vi "CoriEngine.vi"(0 "object in":refnum<class "CoriFlowBFS1Plus.lvclass">, 2 "Sample Rate (Hz)":dbl=10.0 format="%#_13g", 5 "error in (no error)":errorcluster) -> (14 "object out":refnum<class "CoriFlowBFS1Plus.lvclass">, 19 "error out":errorcluster)   [LabVIEW 2021, in "CoriFlowBFS1Plus.lvclass"]
uses:
  CoriFlowBFS1Plus.lvclass
  CoriFlowBFS1Plus.lvclass/CoriFlowBFS1Plus.ctl
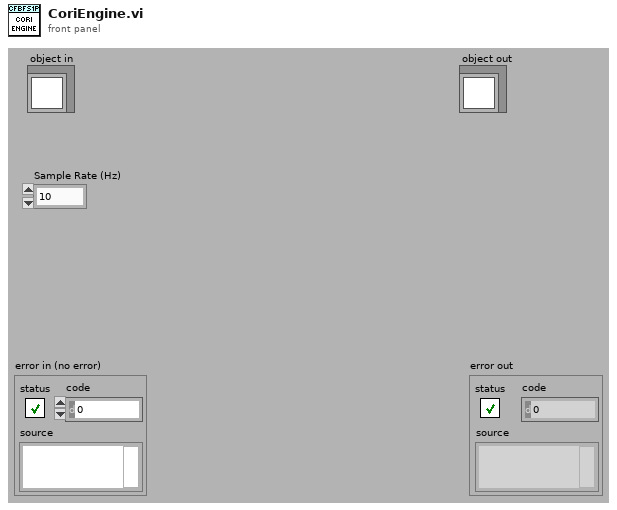
[diagram p1: front panel]
types:
  T1 = cluster{"Message":string, "Message Data":variant}
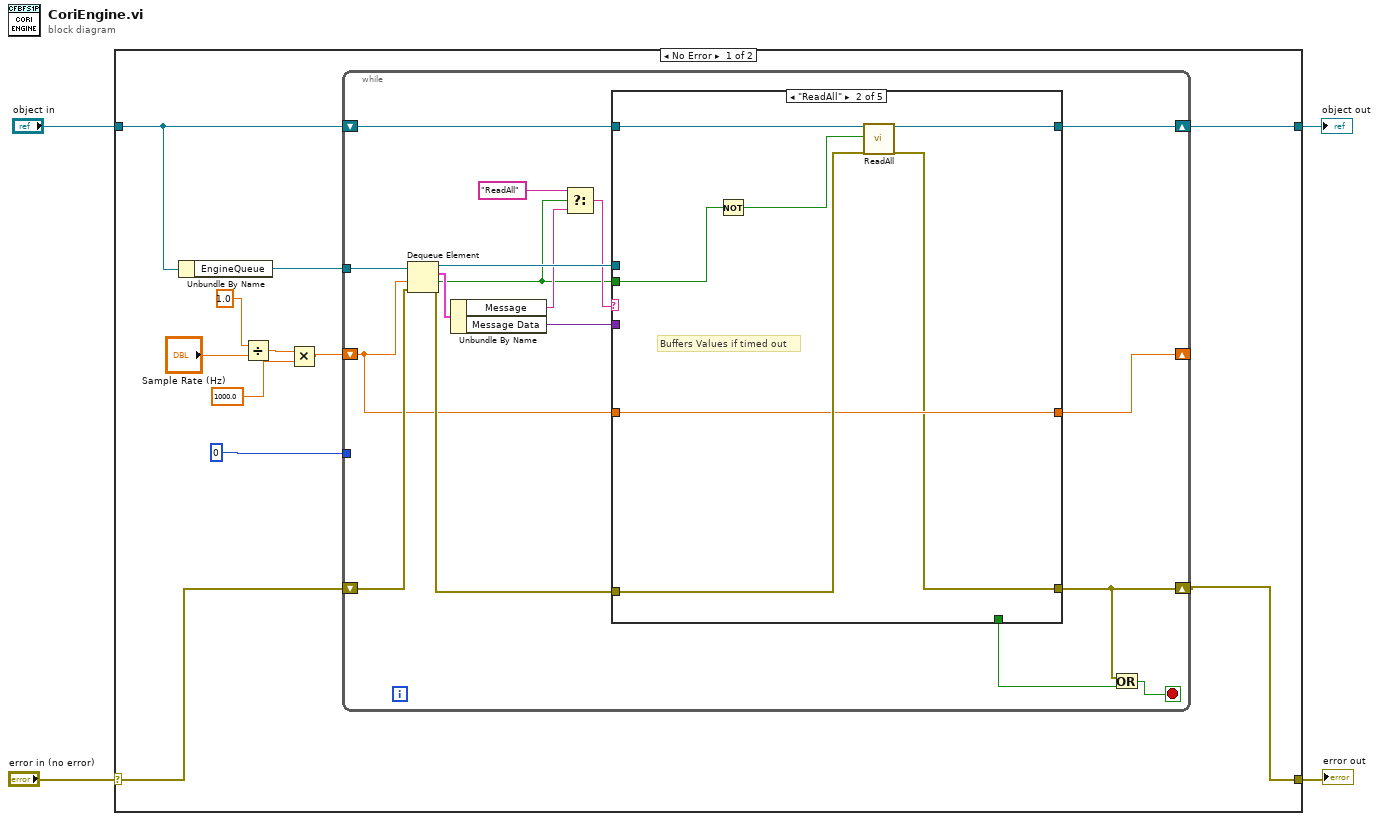
[diagram p0: block diagram]
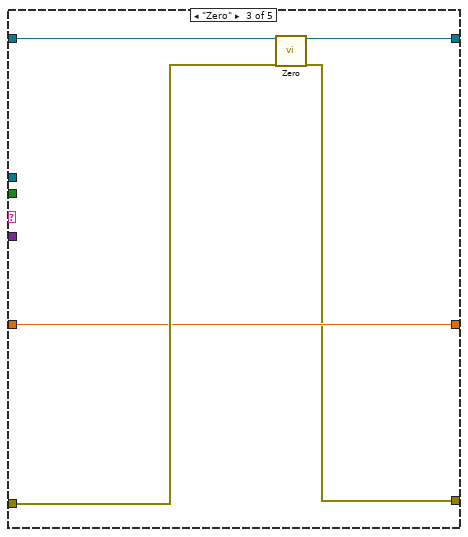
[diagram p3: hidden frame]
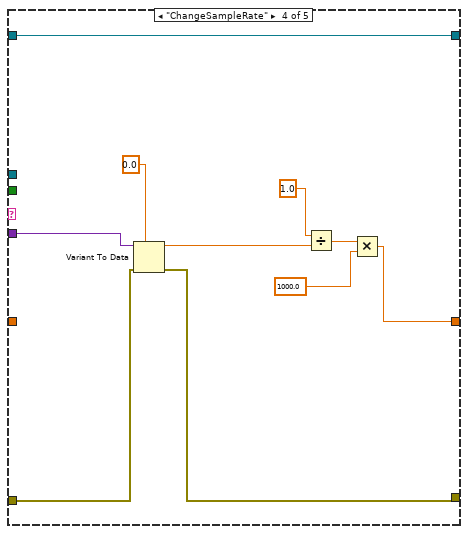
[diagram p4: hidden frame]
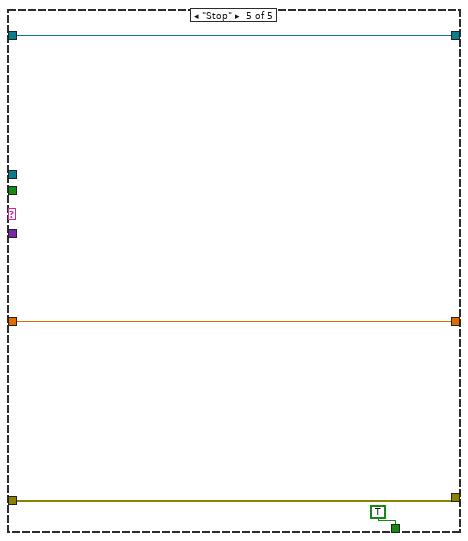
[diagram p5: hidden frame]
diagram:
  n1 = case shown="No Error" "error in (no error)" {
    selector: "error in (no error)" -> [w7 w63]
    tunnel: [w6 w63] -> w3
    tunnel: [w14 w62] -> w1
    tunnel: "object in" -> [w15 w62]
    frame No Error {
      n2 = Unbundle By Name(w15) -> ("EngineQueue"=w5:refnum<queue>)
      n3 = Divide(x=1.0, y="Sample Rate (Hz)") -> (x/y=w10:dbl)
      n4 = Multiply(x=w10, y=1000.0) -> (x*y=w8:dbl)
      n5 = while {
        shift-right: [w24] -> w14
        shift-left: w15 -> [w25]
        tunnel: w5 -> [w32]
        shift-right: [w27] -> w6
        shift-left: w7 -> [w30]
        tunnel: u32 0 ("millisecond multiple") -> [_]
        shift-right: [w23] -> _
        shift-left: w8 -> [w21]
        stop <- w28 stop-if-true
        n6 = Dequeue Element(queue=w32, timeout in ms (-1)=w21, error in (no error)=w30) -> (queue out=w22:refnum<queue>, element=w31:T1, timed out?=w16:bool, error out=w29:errorcluster)
        n7 = Unbundle By Name(w31) -> ("Message"=w18:string, "Message Data"=w17:variant)
        n8 = Select(t="ReadAll", s=w16, f=w18) -> (s? t:f=w20:string)
        n9 = case shown="\"ReadAll\"" w20 {
          tunnel: w22 -> [_ _ _ _ _]
          tunnel: w29 -> [w35 w42 w47 w54 w61]
          tunnel: [w35 w38 w43 w55 w61] -> w27
          tunnel: [_ _ _ _ TRUE] -> w26
          tunnel: [w34 w41 w44 w57 w59] -> w24
          tunnel: w25 -> [w34 w40 w45 w57 w59]
          tunnel: w21 -> [w33 w39 w46 _ w58]
          tunnel: [w33 w39 w46 w49 w58] -> w23
          tunnel: w17 -> [_ _ _ w48 _]
          tunnel: w16 -> [_ w37 _ _ _]
          frame "False", Default {
          }
          frame "ReadAll" {
            # "Buffers Values if timed out"
            n10 = Not(x=w37) -> (.not. x?=w36:bool)
            n11 = call-dynamic "ReadAll.vi"("object in"=w40, "Buffer Values?"=w36, "error in (no error)"=w42) -> ("object out"=w41:refnum<class "CoriFlowBFS1Plus.lvclass">, "error out"=w38:errorcluster)  [unwired: 14 in, 1 out]
          }
          frame "Zero" {
            n12 = call-dynamic "Zero.vi"("object in"=w45, "error in (no error)"=w47) -> ("object out"=w44:refnum<class "CoriFlowBFS1Plus.lvclass">, "error out"=w43:errorcluster)  [unwired: 16 in]
          }
          frame "ChangeSampleRate" {
            n13 = Variant To Data(error in=w54, type=0.0, Variant=w48) -> (data=w50:dbl, error out=w55:errorcluster)
            n14 = Divide(x=1.0, y=w50) -> (x/y=w52:dbl)
            n15 = Multiply(x=w52, y=1000.0) -> (x*y=w49:dbl)
          }
          frame "Stop" {
          }
        }
        n16 = Or(x=w27, y=w26) -> (x .or. y?=w28:bool)
      }
    }
    frame Error {
    }
  }
  "error out" <- w3
  "object out" <- w1
